vi "Unflatten Value.vi"(8 "Error In":errorcluster, 10 "Value":string, 11 "Float In":refnum<class "Flt.lvclass">) -> (0 "Error Out":errorcluster, 3 "Float Out":refnum<class "Flt.lvclass">)   [LabVIEW 2017, in "Tree API.lvlib" / "Flt.lvclass"]
uses:
  Flt.lvclass
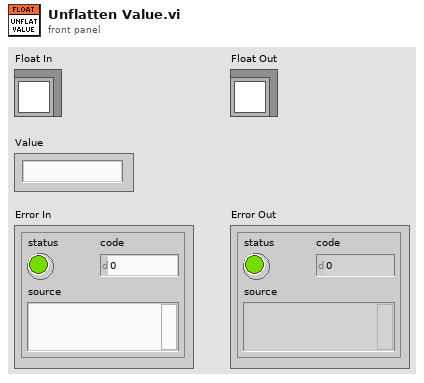
[diagram p1: front panel]
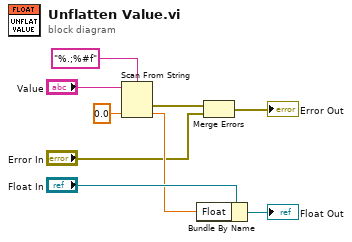
[diagram p0: block diagram]
diagram:
  n1 = Scan From String(format string="%.;%#f" ("initial string"), input string="Value", default 1=0.0 ("default value 1")) -> (error out=w4:errorcluster, output 1=w5:dbl)  [unwired: 2 in, 2 out]
  n2 = Bundle By Name(cluster="Float In", "Float"=w5) -> (→"Float Out":refnum<class "Flt.lvclass">)
  n3 = Merge Errors(w4, "Error In") -> (→"Error Out":errorcluster)
